vi "TDC_DAQV14_after.vi"() -> ()   [LabVIEW 2017]
uses:
  <vilib>/Utility/file.llb/Write Delimited Spreadsheet (DBL).vi
  <vilib>/Utility/file.llb/Write Delimited Spreadsheet (I64).vi
panel:
  in  "display":bool=TRUE
  in  "Thresholds":u16
  in  "one key for threshold":bool
  in  "save data":bool=TRUE
  in  "RST":bool
  out "rate":dbl=7576.957857132235
  in  "Thresholds (mV)":u16[](array[numeric])=[500, 500, 500, 500, 500, 500, 500, 500]
  out "appended path 2":path=path "G:/tdc/2017/test_20230321_035424.csv"
  in  "通道数量":i32=64
  out "Cal Table":u32[](array[numeric])=[0, 0, 0, 100002, 0, 0, 0, 0, 0, 0, 0, 0, 0, 0, 0, 0, 0, 0, 0, 0, 0, 0, 0, 0, 0, 0, 0, 0, 0, 0, 0, 0]
  in  "channel for cal":i32=2
  out "single":u32 format="%08x"
  out "channel number":u64
  in  "bytes to read":i32=80
  out "Calibration Counter":i32=100000
  out "Event index":i32=97959
  out "cal":u32[](graph)
  out "error out":errorcluster
  in  "stop":bool=TRUE
  out "appended path":path=path "G:/tdc/2017/test_20230321_035424.dat"
  in  "filename":string="test"
  in  "Events":i32=110000 min=1
  in  "timeout (ms)":i32=10000
  in  "address":string="192.168.10.10"
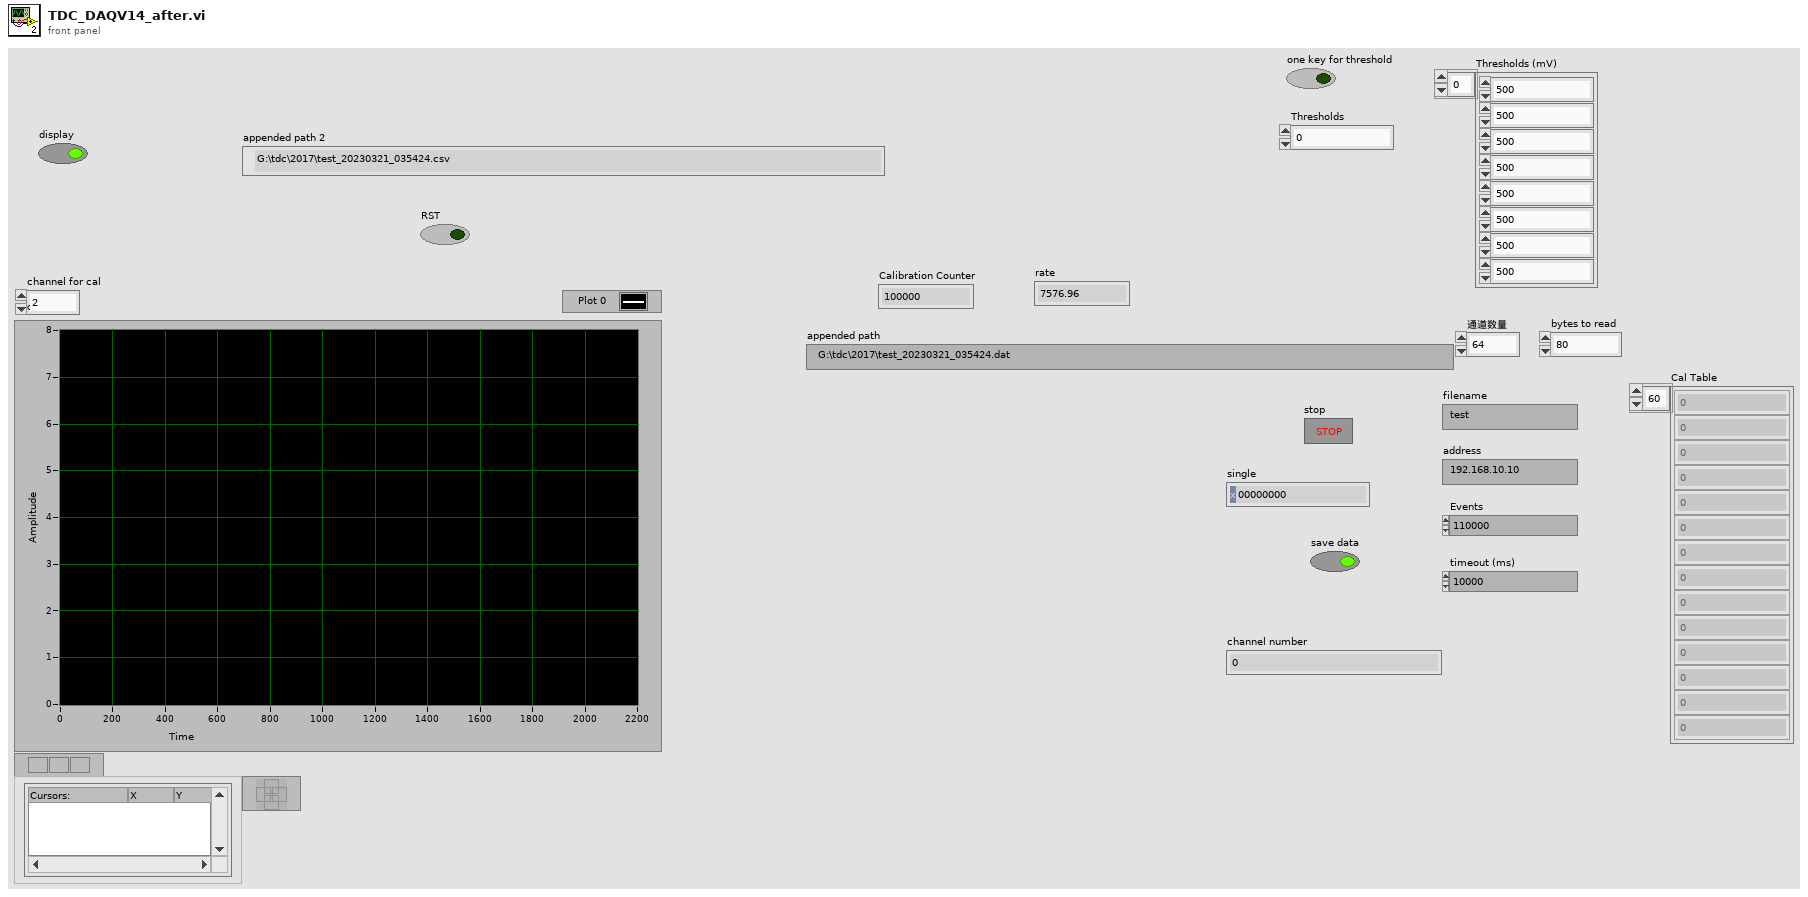
[diagram p1: front panel]
types:
  T1 = enum16{"open", "replace", "create", "open or create", "replace or create", "replace or create with confirmation"}
  T2 = enum16{"big-endian, network order", "native, host order", "little-endian"}
  T3 = enum16{"Standard", "Buffered", "CRLF", "Immediate"}
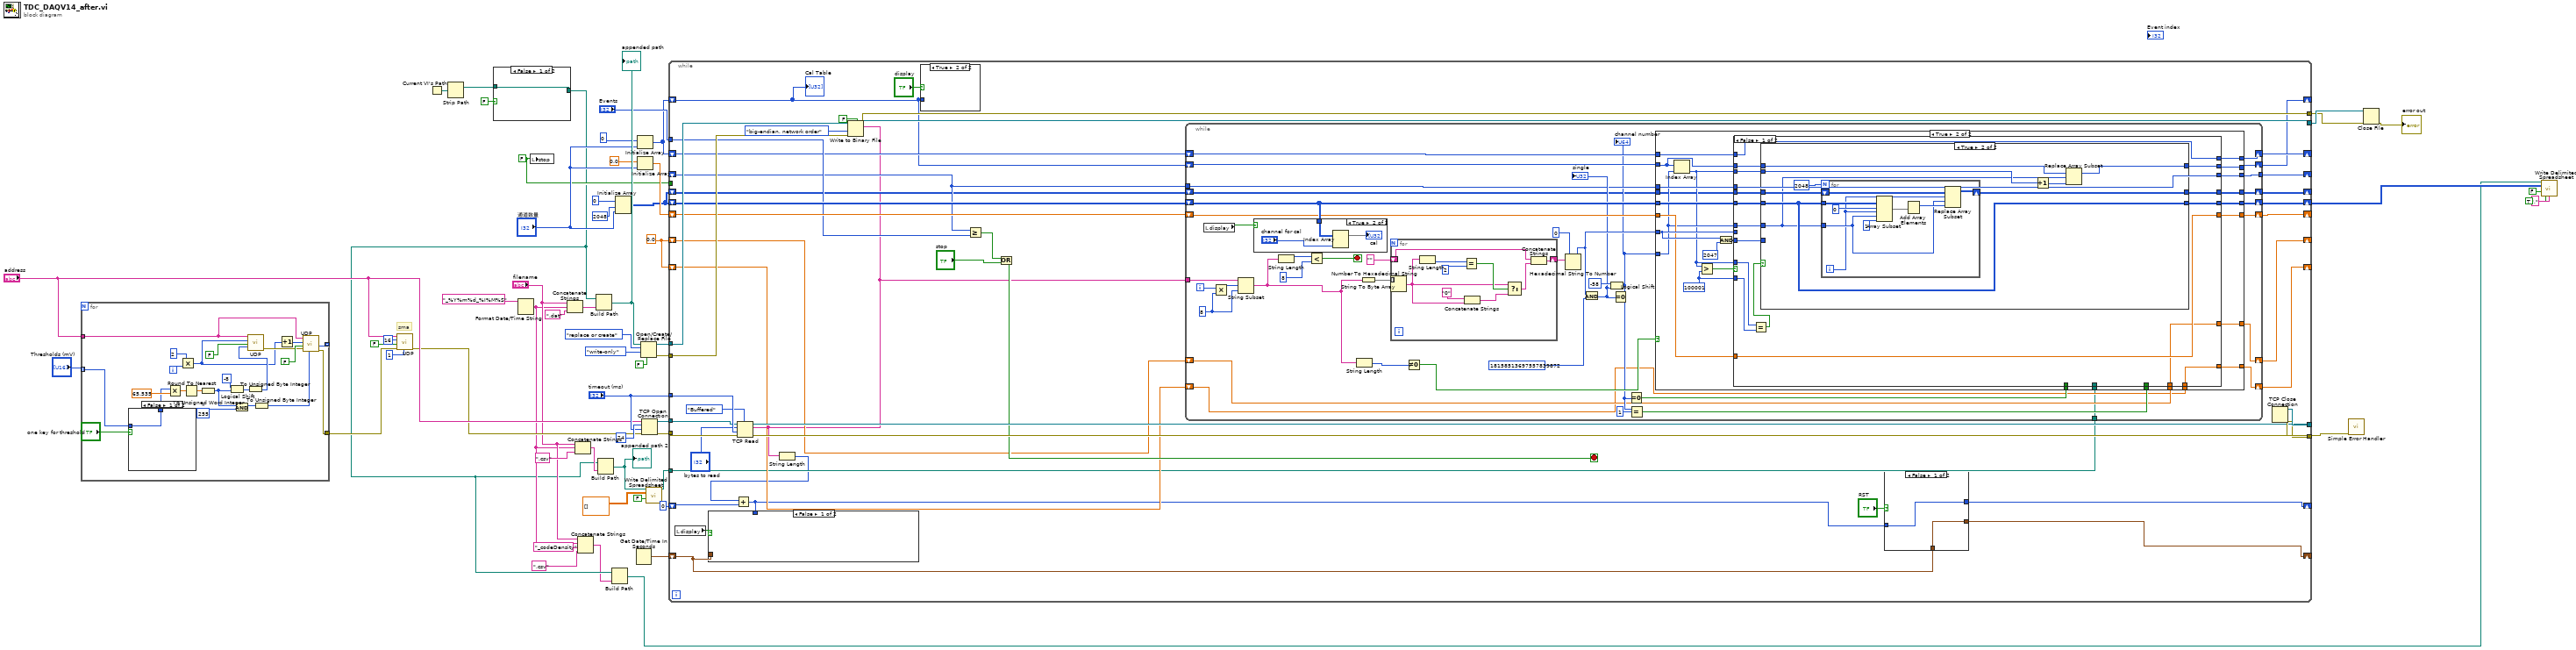
[diagram p0: block diagram]
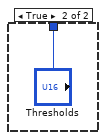
[diagram p2: hidden frame]
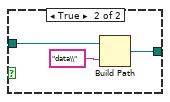
[diagram p3: hidden frame]
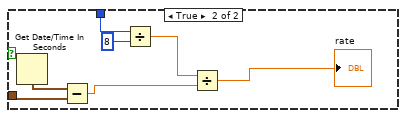
[diagram p4: hidden frame]
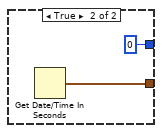
[diagram p6: hidden frame]
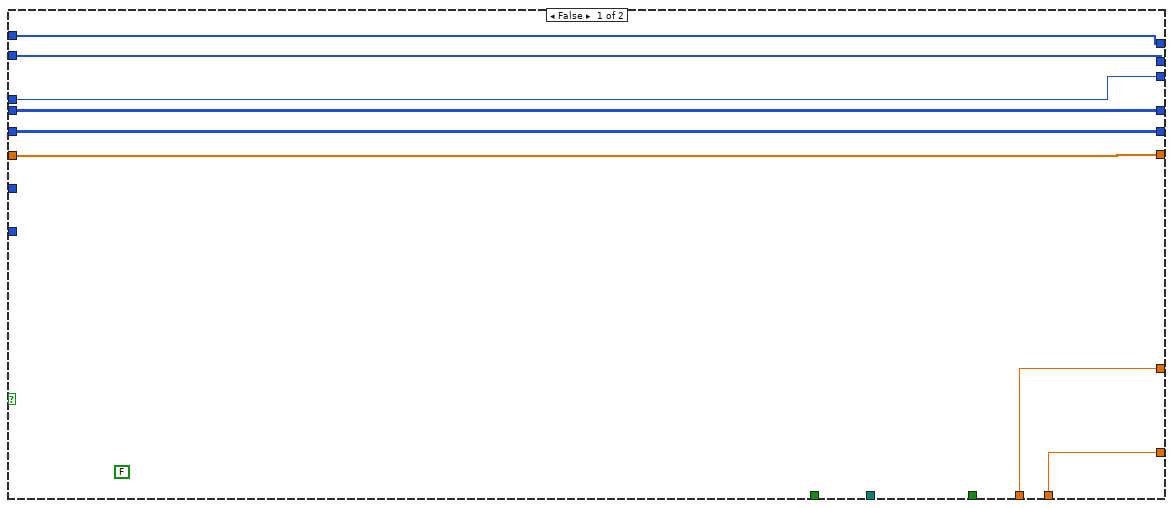
[diagram p8: hidden frame]
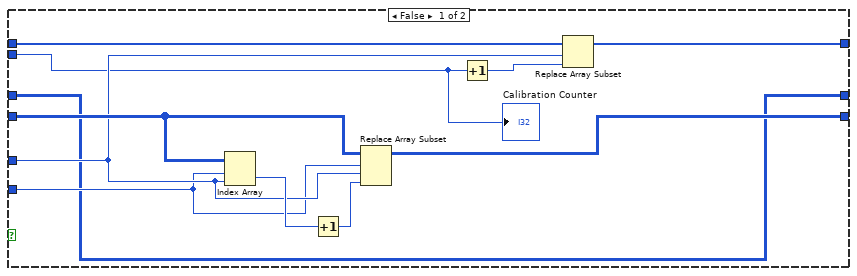
[diagram p9: hidden frame]
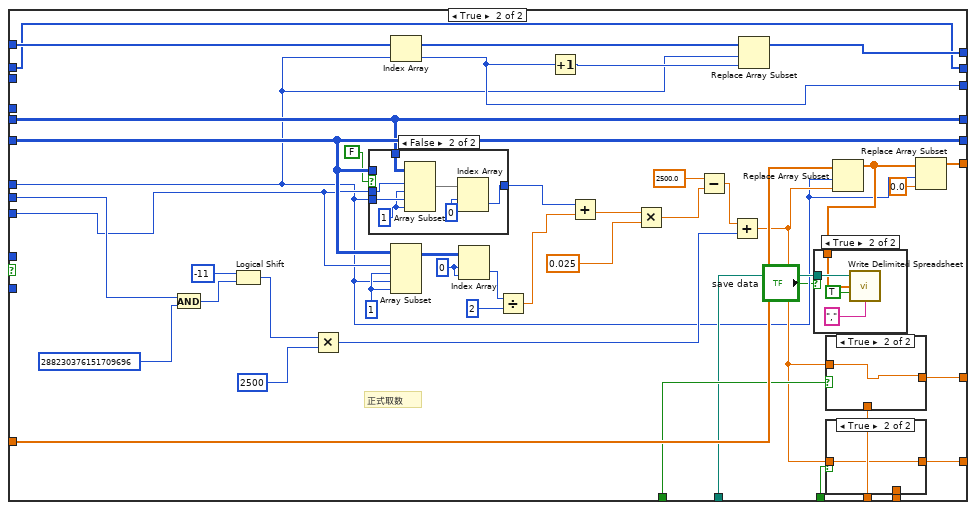
[diagram p10: hidden frame]
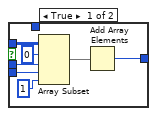
[diagram p12: hidden frame]
diagram:
  w12 = FALSE ("stop")
  w29 = 0.0
  # "sma"
  n1 = for {
    tunnel: "address" -> [w76]
    tunnel: "Thresholds (mV)" -> [w60] mode=indexing
    tunnel: [w69] -> _ mode=indexing
    tunnel: [w63] -> w16
    i -> [w82]
    w71 = u16 255  # x
    n2 = case shown="False" "one key for threshold" {
      tunnel: [w83 "Thresholds"] -> w61
      tunnel: w60 -> [w83 _]
      frame False {
      }
      frame True {
      }
    }
    n3 = Multiply(x=w61, y=65.535) -> (x*y=w79:dbl)
    n4 = Multiply(x=2, y=w82) -> (x*y=w64:i32)
    n5 = Round To Nearest(number=w79) -> (nearest integer value=w77:dbl)
    n6 = To Unsigned Word Integer(number=w77) -> (unsigned 16bit integer=w66:u16)
    n7 = Logical Shift(y=i16 -8, x=w66) -> (x << y=w73:u16)
    n8 = And(x=w66, y=w71) -> (x .and. y?=w70:u16)
    n9 = To Unsigned Byte Integer(number=w73) -> (unsigned 8bit integer=w72:u8)
    n10 = call "UDP.vi"("In"=w72, "Read (TRUE)"=FALSE, "Address"=w64, "IP address"=w76) -> ("error out"=w65:errorcluster)  [unwired: 5 in, 1 out]
    n11 = To Unsigned Byte Integer(number=w70) -> (unsigned 8bit integer=w68:u8)
    n12 = Increment(x=w64) -> (x+1=w75:i32)
    n13 = call "UDP.vi"("In"=w68, "error in (no error)"=w65, "Read (TRUE)"=FALSE, "Address"=w75, "IP address"=w76) -> ("error out"=w63:errorcluster, "Out"=w69:u8)  [unwired: 4 in]
  }
  n14 = call "UDP.vi"("In"=u8 1, "error in (no error)"=w16, "Read (TRUE)"=FALSE, "Address"=u32 16, "IP address"="address") -> ("error out"=w15:errorcluster)  [unwired: 4 in, 1 out]
  n15 = Current VI's Path() -> (path=w49:path)
  n16 = Strip Path(path=w49) -> (stripped path=w48:path)  [unwired: 1 out]
  n17 = case shown="False" FALSE {
    tunnel: w48 -> [w85 w87]
    tunnel: [w85 w86] -> w7
    frame False {
    }
    frame True {
      n18 = Build Path(base path=w87, name or relative path="data\\") -> (appended path=w86:path)
    }
  }
  n19 = Format Date/Time String(time format string (%c)="_%Y%m%d_%I%M%S") -> (date/time string=w10:string)  [unwired: 2 in]
  n20 = local write "stop"(w12) -> ()
  n21 = Concatenate Strings("filename", w10, ".dat") -> (w47:string)
  n22 = Concatenate Strings("filename", w10, ".csv") -> (w31:string)
  n23 = Concatenate Strings("filename", w10, "_codeDensity" ("string"), ".csv") -> (w6:string)
  n24 = Build Path(base path=w7, name or relative path=w47) -> (appended path=w46:path)
  "appended path" <- w46
  n25 = Build Path(base path=w7, name or relative path=w31) -> (appended path=w26:path)
  "appended path 2" <- w26
  n26 = Build Path(base path=w7, name or relative path=w6) -> (appended path=w3:path)
  n27 = Initialize Array(u32 0 ("element"), 2048 ("dimension size"), "通道数量") -> (w28:u32[][])
  n28 = Get Date/Time In Seconds() -> (seconds since 1Jan1904=w19:timestamp)
  n29 = Initialize Array(u32 0 ("element"), "通道数量") -> (w30:u32[])
  n30 = Initialize Array(0.0, "通道数量") -> (w36:dbl[])
  n31 = Open/Create/Replace File(file path (use dialog)=w46, operation (0:open)=T1."replace or create", access (0:read/write)=enum16{"read/write", "read-only", "write-only"}."write-only", disable buffering (F)=FALSE) -> (refnum out=w51:refnum<file>, error out=w50:errorcluster)  [unwired: 2 in, 1 out]
  n32 = TCP Open Connection(address="address", remote port or service name=u16 24 ("port"), timeout ms (60000)="timeout (ms)", error in (no error)=w15) -> (connection ID=w56:refnum<k5>, error out=w55:errorcluster)  [unwired: 1 in]
  n33 = call-poly <vilib>:"Write Delimited Spreadsheet.vi"("file path (dialog if empty)"=w26, "2D data"=dbl[][] [], "append to file? (new file:F)"=FALSE) -> ("new file path (Not A Path if cancelled)"=w25:path)  [unwired: 11 in, 1 out]
  n34 = while {
    tunnel: "timeout (ms)" -> [w132]
    tunnel: w56 -> [w131]
    tunnel: w55 -> [w130]
    tunnel: w51 -> [w125]
    tunnel: w50 -> [w126]
    tunnel: [w128] -> w43
    tunnel: [w127] -> w42
    tunnel: [w124] -> w41
    tunnel: [w123] -> w40
    shift-right: [w119] -> w4
    shift-left: w28 -> [w120]
    shift-right: [w102] -> _
    shift-left: w36 -> [w118]
    tunnel: "Events" -> [w114]
    shift-right: [w113] -> _
    shift-left: w30 -> [w112]
    shift-right: [w111] -> _
    shift-left: _ -> [w110]
    shift-right: [w109] -> _
    shift-left: w30 -> [w89]
    shift-right: [w108] -> _
    shift-left: w29 -> [w105]
    shift-right: [w107] -> _
    shift-left: w29 -> [w106]
    shift-right: [w92] -> _
    shift-left: w28 -> [w104]
    tunnel: w25 -> [w103]
    shift-right: [w96] -> _
    shift-left: 0 -> [w101]
    shift-right: [w94] -> _
    shift-left: w19 -> [w93]
    tunnel: w12 -> [_]
    stop <- w117 stop-if-true
    n35 = local read "display"() -> (w90:bool)
    n36 = TCP Read(connection ID=w131, bytes to read="bytes to read", error in (no error)=w130, 7:T3."Buffered" ("mode (standard)"), 9:w132) -> (connection ID out=w128:refnum<k5>, data out=w99:string, error out=w127:errorcluster)
    n37 = String Length(string=w99) -> (length=w98:i32)
    n38 = Add(x=w98, y=w101) -> (x+y=w97:i32)
    n39 = case shown="False" w90 {
      tunnel: w97 -> [_ w134]
      tunnel: w93 -> [_ w133]
      frame False {
      }
      frame True {
        n40 = Get Date/Time In Seconds() -> (seconds since 1Jan1904=w138:timestamp)
        n41 = Subtract(x=w138, y=w133) -> (x-y=w137:dbl)
        n42 = Divide(x=w134, y=8) -> (x/y=w136:dbl)
        n43 = Divide(x=w136, y=w137) -> (x/y=→"rate":dbl)
      }
    }
    n44 = Write to Binary File(file (use dialog)=w125, data=w99, error in=w126, 5:FALSE ("prepend array or string size? (T)"), 9:T2."big-endian, network order" ("byte order (0:big-endian, network order)")) -> (refnum out=w124:refnum<file>, error out=w123:errorcluster)  [unwired: 1 in, 1 out]
    n45 = case shown="True" "display" {
      tunnel: w89 -> [_ _]
      frame False {
      }
      frame True {
      }
    }
    n46 = Greater Or Equal?(x=w110, y=w114) -> (x >= y?=w115:bool)
    n47 = Or(x=w115, y="stop") -> (x .or. y?=w117:bool)
    n48 = while {
      tunnel: w99 -> [w179]
      shift-right: [w175] -> w119
      shift-left: w120 -> [w173]
      shift-right: [w171] -> w102
      shift-left: w118 -> [w172]
      shift-right: [w165] -> w113
      shift-left: w112 -> [w164]
      tunnel: [w163] -> w111
      tunnel: w110 -> [w162]
      shift-right: [w160] -> w109
      shift-left: w89 -> [w161]
      shift-right: [w152] -> w108
      shift-left: w105 -> [w150]
      shift-right: [w148] -> w107
      shift-left: w106 -> [w149]
      tunnel: w103 -> [w146]
      shift-right: [w145] -> w92
      shift-left: w104 -> [w147]
      i -> [w177]
      stop <- w168 stop-if-true
      w176 = 8 ("length (rest)")
      n49 = local read "display"() -> (w144:bool)
      n50 = Multiply(x=w177, y=w176) -> (x*y=w178:i32)
      n51 = String Subset(string=w179, offset (0)=w178, length (rest)=w176) -> (substring=w159:string)
      n52 = case shown="True" w144 {
        tunnel: w173 -> [_ w186]
        frame False {
        }
        frame True {
          n53 = Index Array(array=w186, index (col)="channel for cal") -> (element=→"cal":u32[])  [unwired: 1 in]
        }
      }
      n54 = String Length(string=w159) -> (length=w170:i32)
      n55 = Less?(x=w170, y=8) -> (x < y?=w168:bool)
      n56 = String Length(string=w159) -> (length=w157:i32)
      n57 = String To Byte Array(string=w159) -> (unsigned byte array=w182:u8[])
      n58 = for {
        shift-right: [w339] -> w181
        shift-left: "" ("format string") -> [w336]
        tunnel: w182 -> [w340] mode=indexing
        n59 = Number To Hexadecimal String(2:w340) -> (0:w332:string)  [unwired: 1 in]
        n60 = String Length(string=w332) -> (length=w338:i32)
        n61 = Equal?(x=w338, y=2) -> (x = y?=w335:bool)
        n62 = Concatenate Strings("0" ("format string"), w332) -> (w334:string)
        n63 = Select(t=w332, s=w335, f=w334) -> (s? t:f=w331:string)
        n64 = Concatenate Strings(w336, w331) -> (w339:string)
      }
      n65 = Not Equal To 0?(x=w157) -> (x != 0?=w156:bool)
      n66 = Hexadecimal String To Number(string=w181, default (0uL)=u64 0 ("default (0 U32)")) -> (number=w174:u64)  [unwired: 1 in, 1 out]
      n67 = And(x=w174, y=u64 18158513697557839872 ("port")) -> (x .and. y?=w166:u64)
      "single" <- w166
      n68 = Logical Shift(y=i16 -58, x=w166) -> (x << y=w155:u64)
      "channel number" <- w155
      n69 = Equal To 0?(x=w166) -> ()  [unwired: 1 out]
      n70 = Equal To 0?(x=w155) -> (x = 0?=w153:bool)
      n71 = Equal?(x=w155, y=u64 1) -> (x = y?=w151:bool)
      n72 = case shown="True" w156 {
        tunnel: w174 -> [_ w220]
        tunnel: w162 -> [w191 w210]
        tunnel: w173 -> [w194 w219]
        tunnel: [w194 w218] -> w175
        tunnel: [w193 w215] -> w171
        tunnel: w172 -> [w193 w214]
        tunnel: w155 -> [_ w209]
        tunnel: w164 -> [w192 w213]
        tunnel: [w192 w212] -> w165
        tunnel: [w191 w211] -> w163
        tunnel: w161 -> [w190 w208]
        tunnel: [w190 w207] -> w160
        tunnel: w153 -> [_ w206]
        tunnel: w150 -> [w189 w205]
        tunnel: [w189 w204] -> w152
        tunnel: w151 -> [_ w203]
        tunnel: w149 -> [w188 w202]
        tunnel: [w188 w201] -> w148
        tunnel: w147 -> [w187 w198]
        tunnel: [w187 w197] -> w145
        tunnel: w146 -> [_ w196]
        frame False {
          (unwired) FALSE
        }
        frame True {
          w199 = 100001 ("y")
          n73 = Index Array(array=w208, index=w209) -> (element=w200:u32)
          n74 = Greater?(x=w200, y=w199) -> (0:w195:bool)
          n75 = And(x=w220, y=u64 2047 ("port")) -> (x .and. y?=w216:u64)
          n76 = case shown="False" w195 {
            tunnel: w220 -> [_ w308]
            tunnel: w219 -> [w237 w290]
            tunnel: [w236 w290] -> w218
            tunnel: w216 -> [w228 w288]
            tunnel: [w235 w271] -> w215
            tunnel: w214 -> [w235 w297]
            tunnel: w210 -> [w233 _]
            tunnel: w209 -> [w231 w269]
            tunnel: w213 -> [w234 w296]
            tunnel: [w234 w295] -> w212
            tunnel: [w233 w293] -> w211
            tunnel: w200 -> [w229 _]
            tunnel: w208 -> [w232 w292]
            tunnel: [w230 w292] -> w207
            tunnel: w206 -> [_ w284]
            tunnel: w205 -> [w227 w283]
            tunnel: [w227 w282] -> w204
            tunnel: w203 -> [_ w281]
            tunnel: w202 -> [w226 w280]
            tunnel: [w226 w279] -> w201
            tunnel: w200 -> [w224 _]
            tunnel: w199 -> [w221 _]
            tunnel: w198 -> [w223 w273]
            tunnel: [w222 w273] -> w197
            tunnel: w196 -> [_ w272]
            frame False {
              n77 = Equal?(x=w224, y=w221) -> (x = y?=w225:bool)
              n78 = case shown="True" w225 {
                tunnel: w237 -> [w248 w254]
                tunnel: [w246 w254] -> w236
                tunnel: w232 -> [w244 w252]
                tunnel: w231 -> [w243 w249]
                tunnel: [w241 w251] -> w230
                tunnel: w229 -> [w240 w250]
                tunnel: w228 -> [w239 _]
                tunnel: w223 -> [w238 w256]
                tunnel: [w238 w255] -> w222
                frame False {
                  n79 = Index Array(array=w248, index (row)=w239, index (col)=w243) -> (element=w247:u32)
                  n80 = Increment(x=w247) -> (x+1=w245:u32)
                  n81 = Replace Array Subset(array=w248, new element=w245, index (row)=w239, index (col)=w243) -> (w246:u32[][])
                  n82 = Increment(x=w240) -> (x+1=w242:u32)
                  n83 = Replace Array Subset(array=w244, new element=w242, index=w243) -> (w241:u32[])
                  "Calibration Counter" <- w240
                }
                frame True {
                  n84 = for {
                    N: 2048 -> [_]
                    tunnel: w254 -> [w266]
                    tunnel: w249 -> [w259]
                    shift-right: [w261] -> w255
                    shift-left: w256 -> [w262]
                    i -> [w258]
                    n85 = Array Subset(array=w266, index (row)=0 ("索引"), length (row)=w258, index (col)=w259, length (col)=1 ("长度")) -> (w263:u32[][])
                    n86 = Add Array Elements(numeric array=w263) -> (sum=w260:u32)
                    n87 = Replace Array Subset(array=w262, new element=w260, index (row)=w258, index (col)=w259) -> (w261:u32[][])
                  }
                  n88 = Increment(x=w250) -> (x+1=w253:u32)
                  n89 = Replace Array Subset(array=w252, new element=w253, index=w249) -> (w251:u32[])
                }
              }
            }
            frame True {
              w286 = 0 ("索引 (行)")
              w289 = 1 ("长度")
              # "正式取数"
              n90 = And(x=w308, y=u64 288230376151709696 ("port")) -> (x .and. y?=w305:u64)
              n91 = Logical Shift(y=i16 -11, x=w305) -> (x << y=w300:u64)
              n92 = Multiply(x=w300, y=u64 2500) -> (x*y=w298:u64)
              n93 = case shown="False" FALSE {
                tunnel: [w314 w321] -> w303
                tunnel: w290 -> [w317 _]
                tunnel: w269 -> [w316 w326]
                tunnel: w288 -> [w315 w324]
                tunnel: w273 -> [_ w325]
                frame True {
                  n94 = Array Subset(array=w317, index (row)=0 ("索引"), length (row)=w315, index (col)=w316, length (col)=1 ("长度")) -> (w318:u32[][])
                  n95 = Add Array Elements(numeric array=w318) -> (sum=w314:u32)
                }
                frame False {
                  w320 = 0 ("index (row)")
                  w323 = 1 ("长度")
                  n96 = Array Subset(array=w325, index (row)=w324, length (row)=w323, index (col)=w326, length (col)=w323) -> (w322:u32[][])
                  n97 = Index Array(array=w322, index (row)=w320, index (col)=w320) -> (element=w321:u32)
                }
              }
              n98 = Index Array(array=w296, index=w269) -> (element=w293:u32)
              n99 = Array Subset(array=w290, index (row)=w288, length (row)=w289, index (col)=w269, length (col)=w289) -> (w287:u32[][])
              n100 = Index Array(array=w287, index (row)=w286, index (col)=w286) -> (element=w285:u32)
              n101 = Divide(x=w285, y=u32 2) -> (x/y=w291:dbl)
              n102 = Increment(x=w293) -> (x+1=w294:u32)
              n103 = Add(x=w303, y=w291) -> (x+y=w302:dbl)
              n104 = Multiply(x=w302, y=0.025) -> (x*y=w276:dbl)
              n105 = Subtract(x=2500.0, y=w276) -> (x-y=w275:dbl)
              n106 = Add(x=w275, y=w298) -> (x+y=w278:dbl)
              n107 = Replace Array Subset(array=w296, new element=w294, index=w269) -> (w295:u32[])
              n108 = case shown="True" w284 {
                tunnel: w278 -> [_ w330]
                tunnel: [w329 w330] -> w282
                tunnel: w283 -> [w329 _]
                frame False {
                }
                frame True {
                }
              }
              n109 = case shown="True" w281 {
                tunnel: [w327 w328] -> w279
                tunnel: w280 -> [w327 _]
                tunnel: w278 -> [_ w328]
                frame False {
                }
                frame True {
                }
              }
              n110 = Replace Array Subset(array=w297, new element=w278, index=w269) -> (w270:dbl[])
              n111 = case shown="True" "save data" {
                tunnel: w272 -> [_ w312]
                tunnel: w270 -> [_ w309]
                frame False {
                }
                frame True {
                  n112 = call-poly <vilib>:"Write Delimited Spreadsheet.vi"("file path (dialog if empty)"=w312, "1D data"=w309, "append to file? (new file:F)"=TRUE, "delimiter (\\t)"="," ("delimiter (\\t)")) -> ()  [unwired: 10 in, 2 out]
                }
              }
              n113 = Replace Array Subset(array=w270, new element=0.0 ("new element/subarray"), index=w269) -> (w271:dbl[])
            }
          }
        }
      }
    }
    n114 = case shown="False" "RST" {
      tunnel: w97 -> [w141 _]
      tunnel: [w141 0] -> w96
      tunnel: [w140 w142] -> w94
      tunnel: w93 -> [w140 _]
      frame False {
      }
      frame True {
        n115 = Get Date/Time In Seconds() -> (seconds since 1Jan1904=w142:timestamp)
      }
    }
    "Cal Table" <- w89
  }
  n116 = TCP Close Connection(connection ID=w43, error in (no error)=w42) -> (error out=w58:errorcluster)  [unwired: 1 in, 1 out]
  n117 = call <vilib>:"Simple Error Handler.vi"("error in (no error)"=w58) -> ()  [unwired: 4 in, 5 out]
  n118 = Close File(refnum=w41, error in=w40) -> (error out=→"error out":errorcluster)  [unwired: 1 out]
  n119 = call-poly <vilib>:"Write Delimited Spreadsheet.vi"("file path (dialog if empty)"=w3, "2D data"=w4, "append to file? (new file:F)"=FALSE, "transpose? (no:F)"=TRUE, "delimiter (\\t)"="," ("delimiter (\\t)")) -> ()  [unwired: 9 in, 2 out]
